vi "Open Log File.vi"(8 "error in (no error)":errorcluster, 10 "Path":path, 11 "PCAP Frame Logger in":refnum<class "PCAP Frame Logger.lvclass">) -> (0 "error out":errorcluster, 3 "PCAP Frame Logger out":refnum<class "PCAP Frame Logger.lvclass">)   [LabVIEW 2020, in "Frame Logging.lvlib" / "PCAP Frame Logger.lvclass"]
uses:
  PCAP Frame Logger.lvclass
  <vilib>/Utility/SystemLogging/NI_SystemLogging.lvlib
  libpcaplv/libpcaplv.lvlib
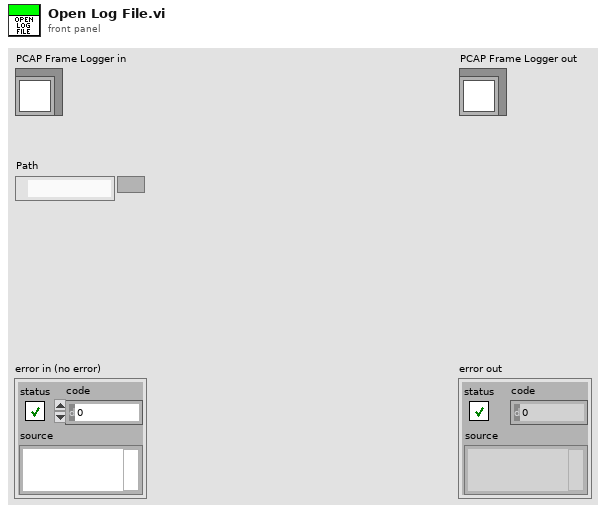
[diagram p1: front panel]
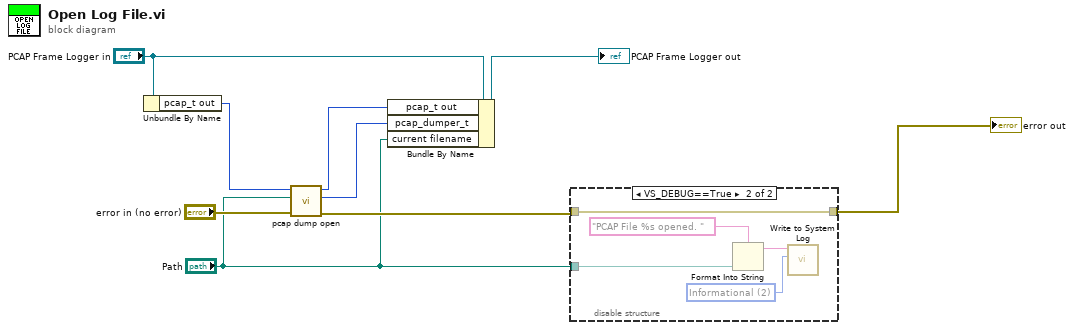
[diagram p0: block diagram]
diagram:
  n1 = Unbundle By Name("PCAP Frame Logger in") -> ("pcap_t out"=w2:u64)
  n2 = call "pcap dump open.vi"("error in"="error in (no error)", "capture file path"="Path", "pcap_t in"=w2) -> ("error out"=w6:errorcluster, "pcap_dumper_t"=w4:u64, "pcap_t out"=w5:u64)  [unwired: 6 in]
  n3 = Bundle By Name(cluster="PCAP Frame Logger in", "pcap_t out"=w5, "pcap_dumper_t"=w4, "current filename"="Path") -> (→"PCAP Frame Logger out":refnum<class "PCAP Frame Logger.lvclass">)
  n4 = disable-structure shown="VS_DEBUG==True" {
    disable-tunnel: w6 -> [_ w11]
    disable-tunnel: [_ w11] -> w9
    disable-tunnel: "Path" -> [_ w10]
    frame condition #0 (active) {
    }
    frame condition #1 {
      w12 = 2 items=["Error", "Warning", "Informational"] ("severity")
      n5 = Format Into String(format string="PCAP File %s opened. ", w10) -> (resulting string=w13:string)  [unwired: 2 in, 1 out]
      n6 = call <vilib>:"Write to System Log.vi"("severity"=w12, "message"=w13) -> ()  [unwired: 9 in, 1 out]
    }
  }
  "error out" <- w9
